vi "Set Resistor.vi"(9 "Set Resistance":T1) -> ()   [LabVIEW 2016]
uses:
  Type_defs/Resistor--enum.ctl
  USB Relay Control 256.vi
panel:
  out "USB":bool
  out "short":bool
  out "0 ohm":bool
  out "100k":bool
  out "10M":bool
  out "Gohm":bool
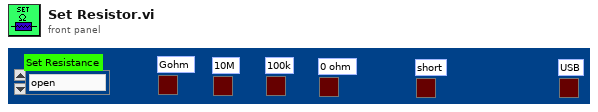
[diagram p1: front panel]
types:
  T1 = typedef "Resistor--enum.ctl" = enum16{"open", "discharge tip", "0 ohms", "100k ohm", "10M ohm", "1G ohm"}
  T2 = enum32{"invalid app kind", "Development System", "Run Time System", "Student Edition", "Embedded LabVIEW", "Evaluation", "Custom"}
  T3 = enum32{"Invalid", "Standard", "Closed", "Hidden", "Minimized", "Maximized"}
  T4 = cluster{"Core":cluster{"Current VI Reference":refnum<vi>, "Close Panel on Exit?":bool}, "Set Resistance":T1, "Previous State":u8, "Intermediate State":u8, "Final State":u8}
  T5 = cluster{"Current VI Reference":refnum<vi>, "Close Panel on Exit?":bool}
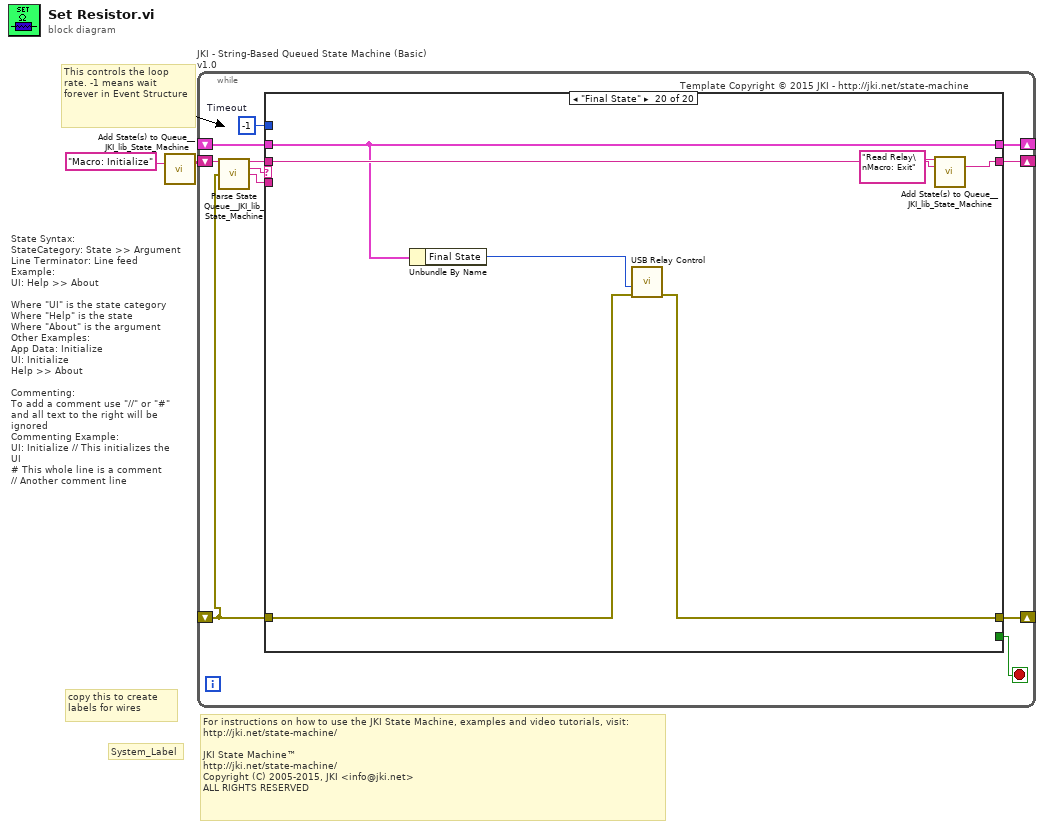
[diagram p0: block diagram]
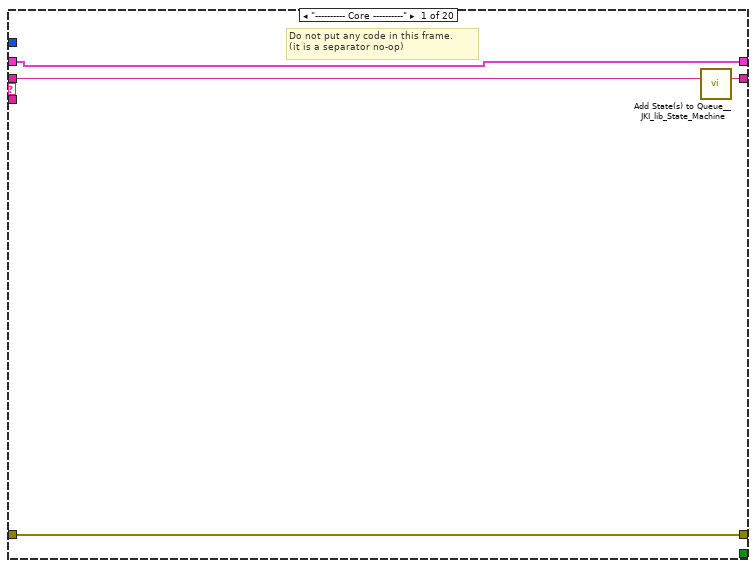
[diagram p2: hidden frame]
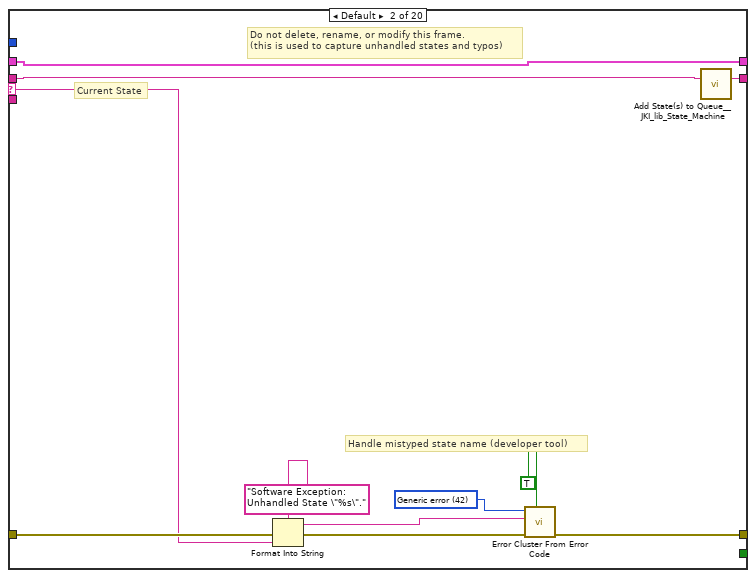
[diagram p3: hidden frame]
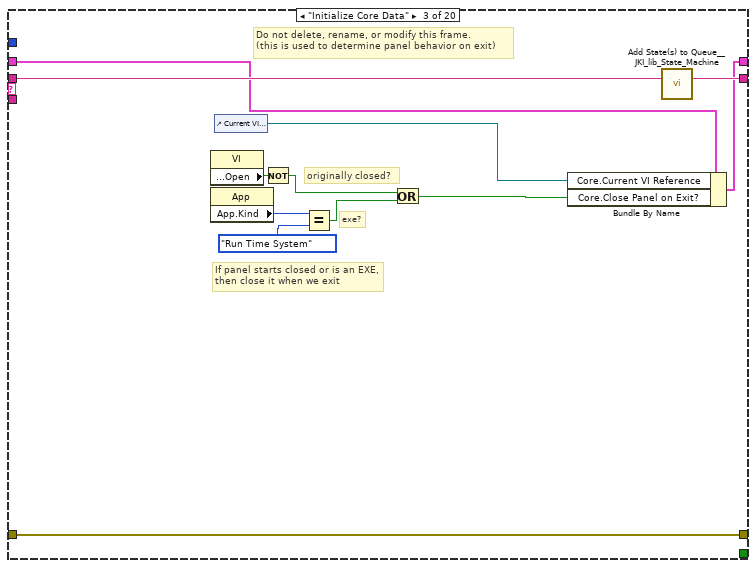
[diagram p4: hidden frame]
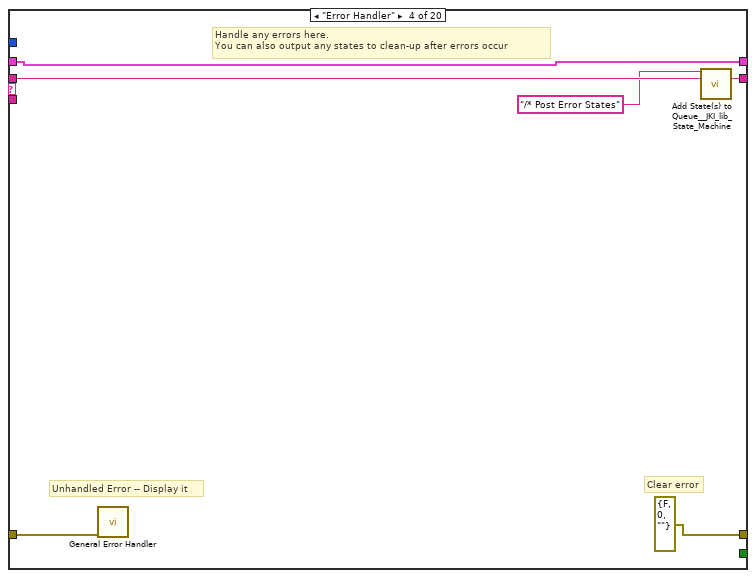
[diagram p5: hidden frame]
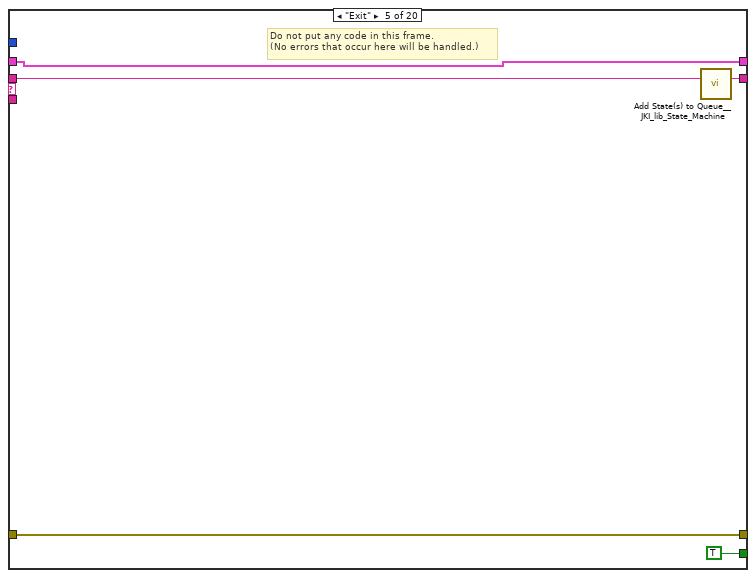
[diagram p6: hidden frame]
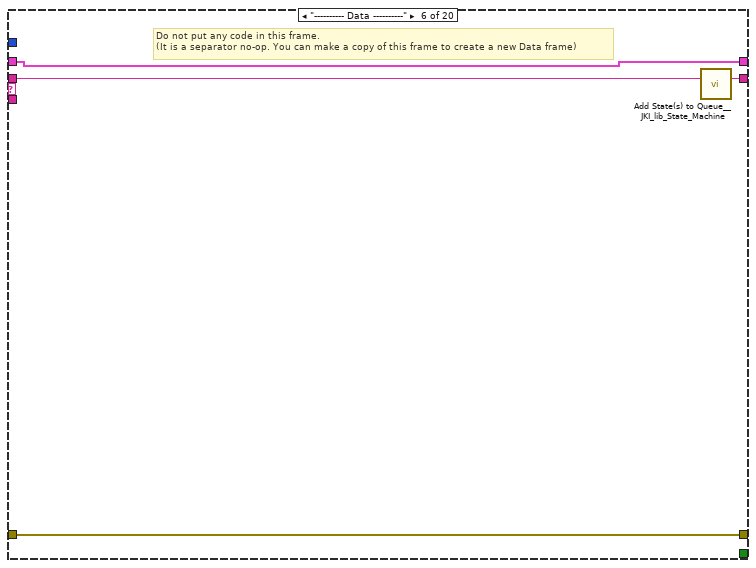
[diagram p7: hidden frame]
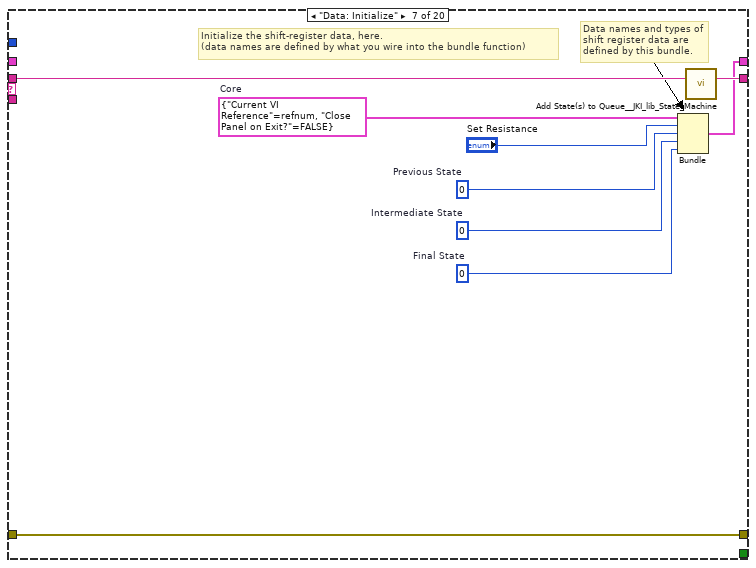
[diagram p8: hidden frame]
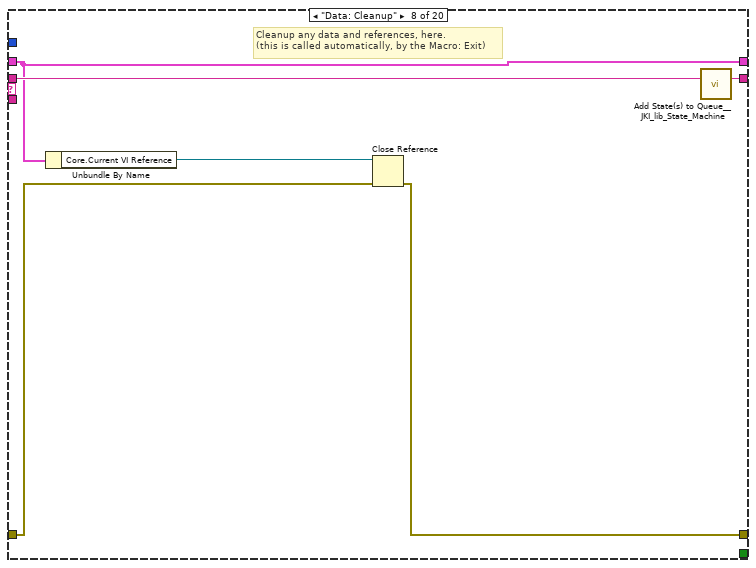
[diagram p9: hidden frame]
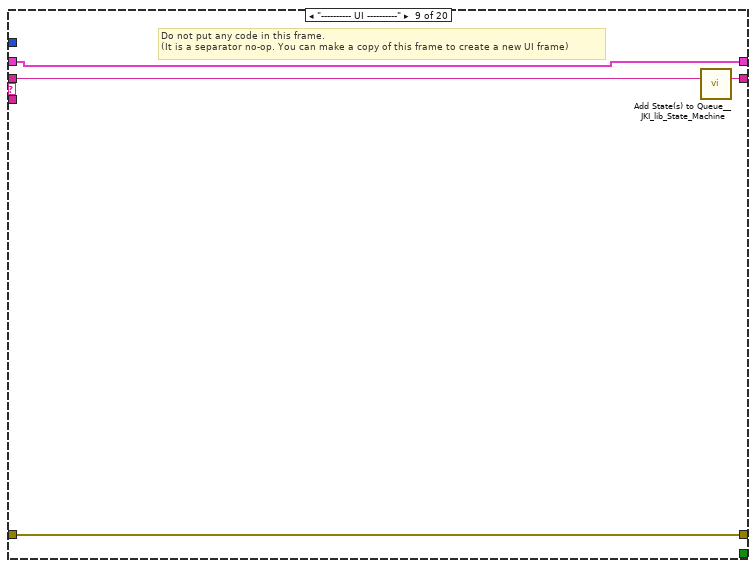
[diagram p10: hidden frame]
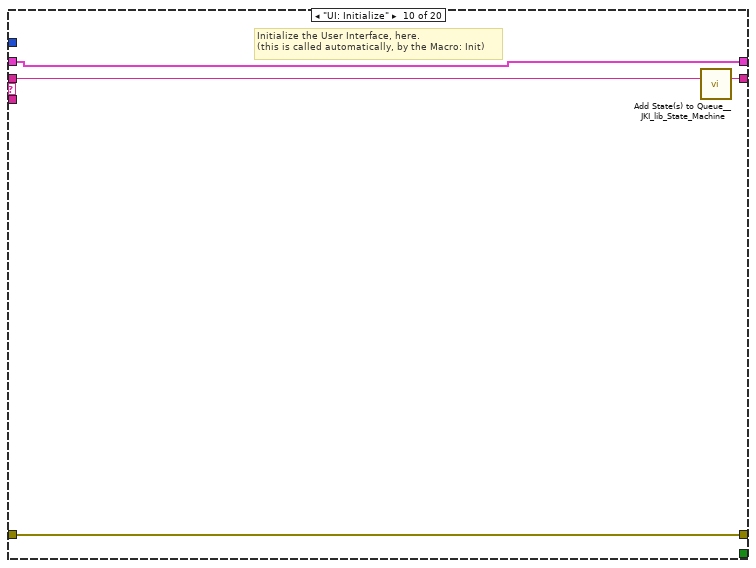
[diagram p11: hidden frame]
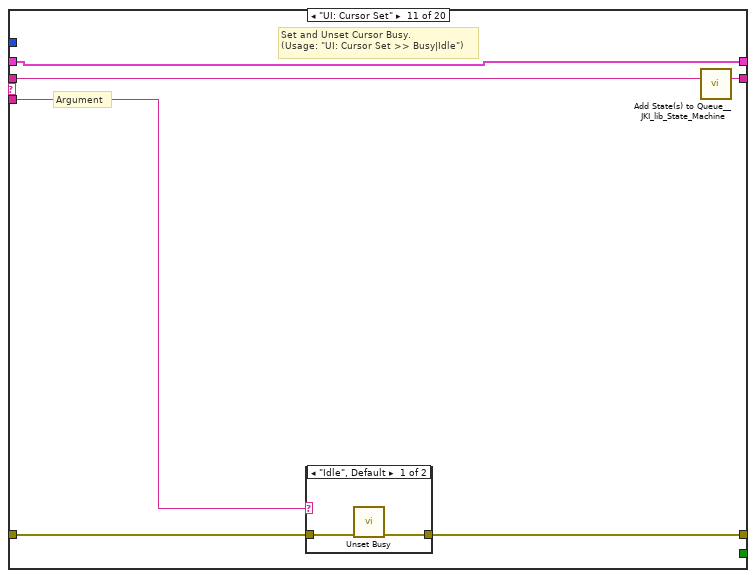
[diagram p12: hidden frame]
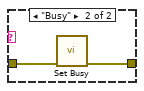
[diagram p13: hidden frame]
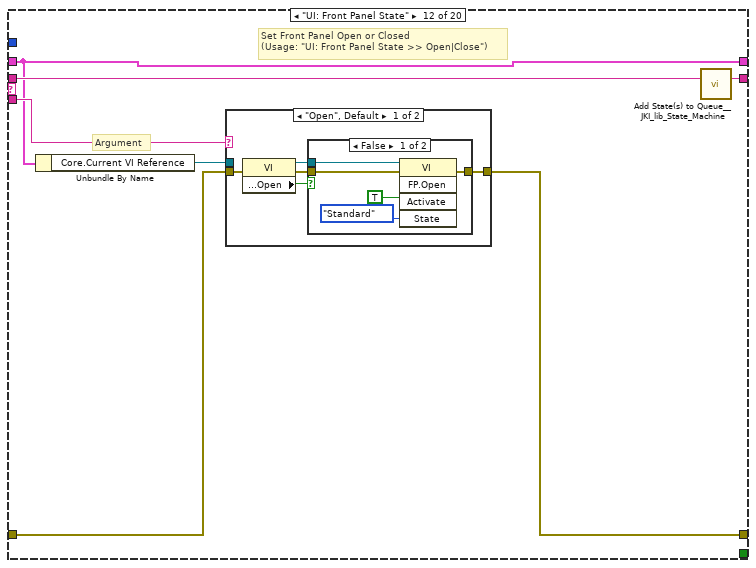
[diagram p14: hidden frame]
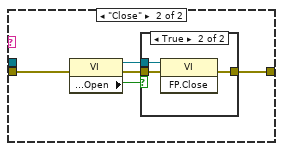
[diagram p16: hidden frame]
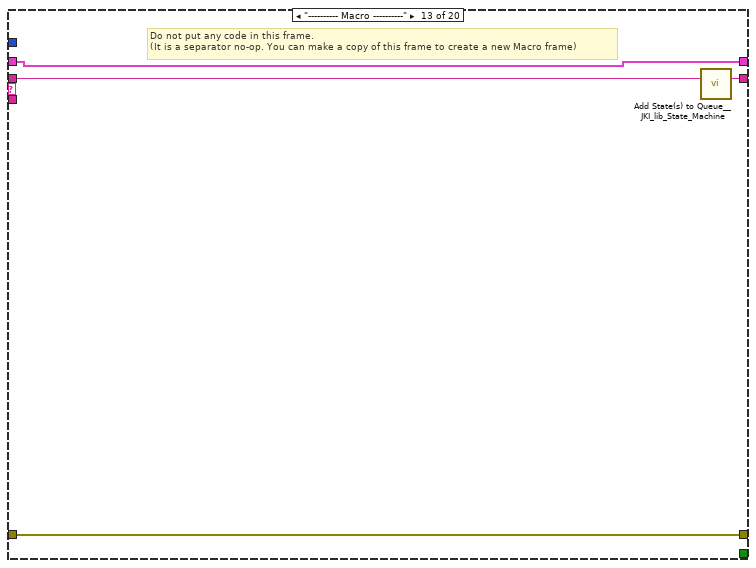
[diagram p18: hidden frame]
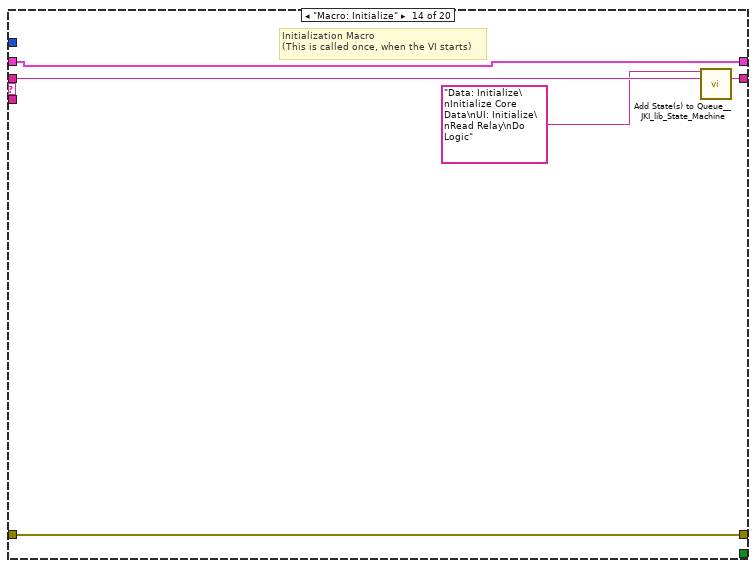
[diagram p19: hidden frame]
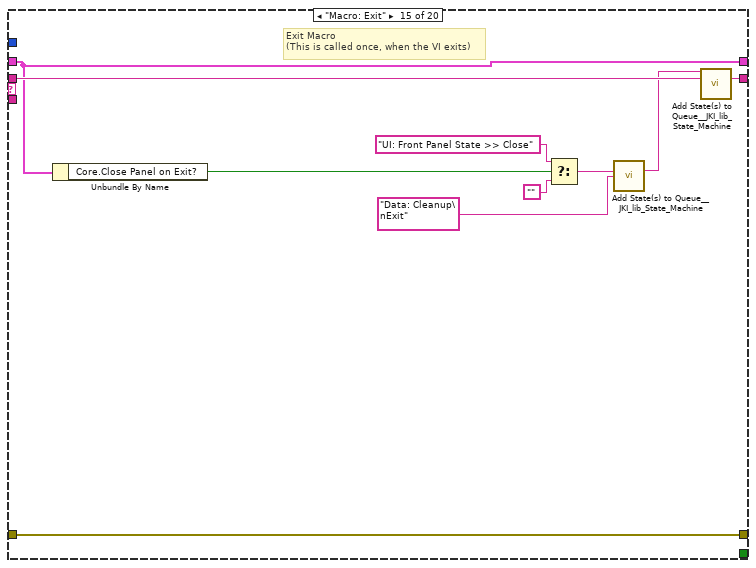
[diagram p20: hidden frame]
diagram:
  # "For instructions on how to use the JKI State Machine, examples and video tutorials, visit:\nhttp://jki.net/state-machine/\n\nJKI State Machine™\nhttp://jki.net/state-machine/\nCopyright (C) 2005-2015, JKI <info@jki.net>\nALL RIGHTS RESERVED"
  # "State Syntax:\nStateCategory: State >> Argument\nLine Terminator: Line feed\nExample:\nUI: Help >> About\n\nWhere \"UI\" is the state category\nWhere \"Help\" is the state\nWhere \"About\" is the argument\nOther Examples:\nApp Data: Initialize\nUI: Initialize\nHelp >> About\n\nCommenting:\nTo add a comment use \"//\" or \"#\" and all text to the right will be ignored\nCommenting Example:\nUI: Initialize // This initializes the UI\n# This whole line is a comment\n// Another comment line"
  # "copy this to create labels for wires"
  # "This controls the loop rate. -1 means wait forever in Event Structure"
  # "System_Label"
  n1 = call <vilib>:"Add State(s) to Queue__JKI_lib_State_Machine.vi"("State(s) in (\"\")"="Macro: Initialize") -> ("States Out"=w2:string)  [unwired: 14 in]
  n2 = while "JKI - String-Based Queued State Machine (Basic) v1.0" {
    shift-right: [w6] -> _
    shift-left: _ -> [w5]
    shift-right: [w9] -> _
    shift-left: _ -> [w3]
    shift-right: [w8] -> _
    shift-left: w2 -> [w10]
    stop <- w7 stop-if-true
    w4 = -1  # Timeout
    # "Template Copyright © 2015 JKI - http://jki.net/state-machine"
    n3 = call <vilib>:"Parse State Queue__JKI_lib_State_Machine.vi"("State Queue"=w10, "Error In (no error)"=w3) -> ("Remaining States"=w12:string, "Current State"=w13:string, "Arguments"=w11:string)  [unwired: 11 in]
    n4 = case shown="\"Final State\"" w13 {
      selector: w13 -> [_ w18 _ _ _ _ _ _ _ _ _ _ _ _ _ _ _ _ _ _]
      tunnel: w12 -> [w17 w22 w40 w46 w51 w55 w64 w70 w74 w78 w84 w95 w119 w124 w134 w138 w156 w169 w287 w294]
      tunnel: w11 -> [_ _ _ _ _ _ _ _ _ _ w79 w90 _ _ _ _ _ _ _ _]
      tunnel: w5 -> [w14 w20 w29 w43 w49 w52 _ w66 w71 w76 w82 w89 w116 w121 w126 w135 w153 w162 w285 w292]
      tunnel: [w15 w24 w38 errorcluster {"status"=FALSE, "code"=0, "source"=""} ("error out") w48 w53 w62 w67 w72 w75 w80 w92 w117 w122 w132 w136 w154 w167 w284 w290] -> w9
      tunnel: w3 -> [w15 w23 w38 w42 w48 w53 w62 w68 w72 w75 w81 w93 w117 w122 w132 w136 w154 w167 w283 w291]
      tunnel: [w16 w21 w39 w45 w50 w54 w63 w69 w73 w77 w83 w94 w118 w123 w133 w137 w155 w168 w288 w295] -> w8
      tunnel: [_ _ _ _ TRUE _ _ _ _ _ _ _ _ _ _ _ _ _ _ _] -> w7
      tunnel: [w14 w20 w30 w43 w49 w52 w59 w66 w71 w76 w82 w89 w116 w121 w126 w135 w152 w161 w285 w292] -> w6
      tunnel: w4 -> [_ _ _ _ _ _ _ _ _ _ _ _ _ _ _ _ _ _ _ _]
      frame "---------- Core ----------" {
        # "Do not put any code in this frame.\n(it is a separator no-op)"
        n5 = call <vilib>:"Add State(s) to Queue__JKI_lib_State_Machine.vi"("State(s) in (\"\")"=w17) -> ("States Out"=w16:string)  [unwired: 14 in]
      }
      frame Default {
        w27 = 42 items=["No error", "Argument error", "Memory is full", "Out of zone", "End of file", "File already open", "Generic file I/O error", "File not found", "File permission error", "Disk is full", "Duplicate path", "Too many files open", "System feature not enabled", "Resource file not found", "Cannot add resource", "Resource not found", "Image not found", "Image memory error", "Pen does not exist", "Config type invalid", "Config token not found", "Config parse error", "Config memory error", "Bad external code format", "Bad external code offset", "External code not present", "Null window", "Destroy window error", "Null menu", "Print aborted", "Bad print record", "Print driver error", "Windows error during printing", "Memory error during printing", "Print dialog error", "Generic print error", "Invalid device refnum", "Device not found", "Device parameter error", "Device unit error", "Cannot open device", "Device call aborted", "Generic error", "Cancelled by user", "Object ID too low", "Object ID too high", "Object not in heap", "Unknown heap", "Unknown object (invalid DefProc)", "Unknown object (DefProc not in table)", "Message out of range", "Invalid (null) method", "Unknown message", "Manager call not supported", "Bad address", "Network operation in progress", "Network operation timed out", "Connection is busy", "Network attribute not supported", "Network error", "Address in use", "System out of memory", "Connection aborted", "Connection refused", "Not connected", "Already connected", "Connection closed", "Initialization error (interapplication manager)", "Bad occurrence", "Wait on unbound occurrence handler", "Occurrence queue overflow", "Datalog type conflict", "Unused", "Unrecognized type (interapplication manager)", "Memory corrupt", "Failed to make temporary DLL", "Old CIN version", "Drag socket not found", "Failed to load drop-object", "Failed to register OLE object", "Failed to release OLE object", "Format specifier type mismatch", "Unknown format specifier", "Too few format specifiers", "Too many format specifiers", "Scan failed", "Newer CIN version", "Error converting to variant", "Runtime menu error", "Password tampered", "Variant attribute not found", "Incompatible variant data type", "Event data is not available", "Event Store is not present", "Occurrence is not found", "Event Queue is not created", "Event info is not available", "Refnum passed is NULL", "Error retrieving Class GUID", "Error retrieving CoClass GUID", "Error retrieving TypeLib GUID.", "Bad built application magic bytes.", "Specific driver is different from the specific driver associated with the Logical Name.", "There is no session opened to the class driver.", "Max Error", "MAX - Error with config objects", "MAX - Error loading configuration", "MAX - Group not supported"]
        # "Current State"
        # "Do not delete, rename, or modify this frame.\n(this is used to capture unhandled states and typos)"
        # "Handle mistyped state name (developer tool)"
        n6 = Format Into String(format string="Software Exception: Unhandled State \"%s\"." ("message"), error in=w23, w18) -> (resulting string=w26:string, error out=w25:errorcluster)  [unwired: 1 in]
        n7 = call <vilib>:"Error Cluster From Error Code.vi"("show call chain? (False)"=TRUE, "error in (no error)"=w25, "error message (\"\")"=w26, "error code (0)"=w27) -> ("error out"=w24:errorcluster)  [unwired: 5 in]
        n8 = call <vilib>:"Add State(s) to Queue__JKI_lib_State_Machine.vi"("State(s) in (\"\")"=w22) -> ("States Out"=w21:string)  [unwired: 14 in]
      }
      frame "Initialize Core Data" {
        # "Do not delete, rename, or modify this frame.\n(this is used to determine panel behavior on exit)"
        # "originally closed?"
        # "exe?"
        # "If panel starts closed or is an EXE, then close it when we exit"
        n9 = property class="VI"() -> ("Front Panel.Open"=w37:bool)  [unwired: 2 in, 2 out]
        n10 = property class="App"() -> ("App.Kind"=w36:T2)  [unwired: 2 in, 2 out]
        n11 = control-ref of="Current VI Reference"() -> (w31:refnum<vi>)
        n12 = Not(x=w37) -> (.not. x?=w34:bool)
        n13 = Equal?(x=w36, y=T2."Run Time System" ("Application:Kind")) -> (x = y?=w33:bool)
        n14 = Or(x=w34, y=w33) -> (x .or. y?=w32:bool)
        n15 = Bundle By Name(cluster=w29, "Core.Current VI Reference"=w31, "Core.Close Panel on Exit?"=w32) -> (w30:T4)
        n16 = call <vilib>:"Add State(s) to Queue__JKI_lib_State_Machine.vi"("State(s) in (\"\")"=w40) -> ("States Out"=w39:string)  [unwired: 14 in]
      }
      frame "Error Handler" {
        # "Unhandled Error -- Display it"
        # "Handle any errors here.\nYou can also output any states to clean-up after errors occur"
        # "Clear error"
        n17 = call <vilib>:"General Error Handler.vi"("error in (no error)"=w42) -> ()  [unwired: 10 in, 5 out]
        n18 = call <vilib>:"Add State(s) to Queue__JKI_lib_State_Machine.vi"("State(s) in Front (\"\")"="/* Post Error States", "State(s) in (\"\")"=w46) -> ("States Out"=w45:string)  [unwired: 13 in]
      }
      frame "Exit" {
        # "Do not put any code in this frame.\n(No errors that occur here will be handled.)"
        n19 = call <vilib>:"Add State(s) to Queue__JKI_lib_State_Machine.vi"("State(s) in (\"\")"=w51) -> ("States Out"=w50:string)  [unwired: 14 in]
      }
      frame "---------- Data ----------" {
        # "Do not put any code in this frame.\n(It is a separator no-op. You can make a copy of this frame to create a new Data frame)"
        n20 = call <vilib>:"Add State(s) to Queue__JKI_lib_State_Machine.vi"("State(s) in (\"\")"=w55) -> ("States Out"=w54:string)  [unwired: 14 in]
      }
      frame "Data: Initialize" {
        w56 = u8 0  # Final State
        w57 = u8 0  # Intermediate State
        w58 = u8 0  # Previous State
        w61 = T5 {"Current VI Reference"=refnum, "Close Panel on Exit?"=FALSE}  # Core
        # "Data names and types of shift register data are defined by this bundle."
        # "Initialize the shift-register data, here.\n(data names are defined by what you wire into the bundle function)"
        n21 = Bundle("Core"=w61, "Set Resistance"="Set Resistance", "Previous State"=w58, "Intermediate State"=w57, "Final State"=w56) -> (w59:T4)  [unwired: 1 in]
        n22 = call <vilib>:"Add State(s) to Queue__JKI_lib_State_Machine.vi"("State(s) in (\"\")"=w64) -> ("States Out"=w63:string)  [unwired: 14 in]
      }
      frame "Data: Cleanup" {
        # "Cleanup any data and references, here.\n(this is called automatically, by the Macro: Exit)"
        n23 = Unbundle By Name(w66) -> ("Core.Current VI Reference"=w65:refnum<vi>)
        n24 = Close Reference(reference=w65, error in (no error)=w68) -> (error out=w67:errorcluster)
        n25 = call <vilib>:"Add State(s) to Queue__JKI_lib_State_Machine.vi"("State(s) in (\"\")"=w70) -> ("States Out"=w69:string)  [unwired: 14 in]
      }
      frame "---------- UI ----------" {
        # "Do not put any code in this frame.\n(It is a separator no-op. You can make a copy of this frame to create a new UI frame)"
        n26 = call <vilib>:"Add State(s) to Queue__JKI_lib_State_Machine.vi"("State(s) in (\"\")"=w74) -> ("States Out"=w73:string)  [unwired: 14 in]
      }
      frame "UI: Initialize" {
        # "Initialize the User Interface, here.\n(this is called automatically, by the Macro: Init)"
        n27 = call <vilib>:"Add State(s) to Queue__JKI_lib_State_Machine.vi"("State(s) in (\"\")"=w78) -> ("States Out"=w77:string)  [unwired: 14 in]
      }
      frame "UI: Cursor Set" {
        # "Argument"
        # "Set and Unset Cursor Busy.\n(Usage: \"UI: Cursor Set >> Busy|Idle\")"
        n28 = case shown="\"Idle\", Default" w79 {
          tunnel: w81 -> [w86 w88]
          tunnel: [w85 w87] -> w80
          frame "Idle", Default {
            n29 = call <vilib>:"Unset Busy.vi"("error in (no error)"=w86) -> ("error out"=w85:errorcluster)  [unwired: 10 in]
          }
          frame "Busy" {
            n30 = call <vilib>:"Set Busy.vi"("error in (no error)"=w88) -> ("error out"=w87:errorcluster)  [unwired: 9 in, 1 out]
          }
        }
        n31 = call <vilib>:"Add State(s) to Queue__JKI_lib_State_Machine.vi"("State(s) in (\"\")"=w84) -> ("States Out"=w83:string)  [unwired: 14 in]
      }
      frame "UI: Front Panel State" {
        # "Argument"
        # "Set Front Panel Open or Closed\n(Usage: \"UI: Front Panel State >> Open|Close\")"
        n32 = Unbundle By Name(w89) -> ("Core.Current VI Reference"=w91:refnum<vi>)
        n33 = case shown="\"Open\", Default" w90 {
          tunnel: w93 -> [w99 w110]
          tunnel: [w100 w111] -> w92
          tunnel: w91 -> [_ _]
          frame "Open", Default {
            n34 = property class="VI"(error in=w99) -> (reference out=w97:refnum<vi>, error out=w98:errorcluster, "Front Panel.Open"=w96:bool)  [unwired: 1 in]
            n35 = case shown="False" w96 {
              tunnel: [w103 w106] -> w100
              tunnel: w98 -> [w102 w106]
              tunnel: w97 -> [w101 _]
              frame False {
                n36 = invoke class="VI" method="FP.Open"(reference=w101, error in=w102, "Activate"=TRUE, "State"=T3."Standard") -> (error out=w103:errorcluster)  [unwired: 1 in, 4 out]
              }
              frame True {
              }
            }
          }
          frame "Close" {
            n37 = property class="VI"(error in=w110) -> (reference out=w108:refnum<vi>, error out=w109:errorcluster, "Front Panel.Open"=w107:bool)  [unwired: 1 in]
            n38 = case shown="True" w107 {
              tunnel: [w112 w115] -> w111
              tunnel: w109 -> [w112 w114]
              tunnel: w108 -> [_ w113]
              frame False {
              }
              frame True {
                n39 = invoke class="VI" method="FP.Close"(reference=w113, error in=w114) -> (error out=w115:errorcluster)  [unwired: 1 in, 2 out]
              }
            }
          }
        }
        n40 = call <vilib>:"Add State(s) to Queue__JKI_lib_State_Machine.vi"("State(s) in (\"\")"=w95) -> ("States Out"=w94:string)  [unwired: 14 in]
      }
      frame "---------- Macro ----------" {
        # "Do not put any code in this frame.\n(It is a separator no-op. You can make a copy of this frame to create a new Macro frame)"
        n41 = call <vilib>:"Add State(s) to Queue__JKI_lib_State_Machine.vi"("State(s) in (\"\")"=w119) -> ("States Out"=w118:string)  [unwired: 14 in]
      }
      frame "Macro: Initialize" {
        # "Initialization Macro\n(This is called once, when the VI starts)"
        n42 = call <vilib>:"Add State(s) to Queue__JKI_lib_State_Machine.vi"("State(s) in Front (\"\")"="Data: Initialize\nInitialize Core Data\nUI: Initialize\nRead Relay\nDo Logic", "State(s) in (\"\")"=w124) -> ("States Out"=w123:string)  [unwired: 13 in]
      }
      frame "Macro: Exit" {
        # "Exit Macro\n(This is called once, when the VI exits)"
        n43 = Unbundle By Name(w126) -> ("Core.Close Panel on Exit?"=w125:bool)
        n44 = Select(t="UI: Front Panel State >> Close", s=w125, f="") -> (s? t:f=w129:string)
        n45 = call <vilib>:"Add State(s) to Queue__JKI_lib_State_Machine.vi"("State(s) in (\"\")"=w129, "State(s) at Back (\"\")"="Data: Cleanup\nExit") -> ("States Out"=w127:string)  [unwired: 13 in]
        n46 = call <vilib>:"Add State(s) to Queue__JKI_lib_State_Machine.vi"("State(s) in Front (\"\")"=w127, "State(s) in (\"\")"=w134) -> ("States Out"=w133:string)  [unwired: 13 in]
      }
      frame "---------- Relay ----------" {
        # "Template Separator\n(You can make a copy of, or modify, this frame)"
        n47 = call <vilib>:"Add State(s) to Queue__JKI_lib_State_Machine.vi"("State(s) in (\"\")"=w138) -> ("States Out"=w137:string)  [unwired: 14 in]
      }
      frame "Read Relay" {
        # "Your code here.\n(You can make a copy of, or modify, this frame)"
        n48 = call "Read_relay.vi"() -> ("unsigned 8bit integer"=w151:u8, "Boolean array"=w145:bool[])  [unwired: 1 in]
        n49 = Index Array(array=w145, index=7) -> (element=→"Gohm":bool)
        n50 = Index Array(array=w145, index=6) -> (element=→"10M":bool)
        n51 = Index Array(array=w145, index=5) -> (element=→"100k":bool)
        n52 = Index Array(array=w145, index=3) -> (element=→"0 ohm":bool)
        n53 = Index Array(array=w145, index=1) -> (element=→"short":bool)
        n54 = Bundle By Name(cluster=w153, "Previous State"=w151) -> (w152:T4)
        n55 = call <vilib>:"Add State(s) to Queue__JKI_lib_State_Machine.vi"("State(s) in (\"\")"=w156) -> ("States Out"=w155:string)  [unwired: 14 in]
        "USB" <- TRUE ("USB")
      }
      frame "Do Logic" {
        # "Your code here.\n(You can make a copy of, or modify, this frame)"
        n56 = Unbundle By Name(w162) -> ("Set Resistance"=w166:T1, "Previous State"=w157:u8)
        n57 = case shown="\"discharge tip\"" w166 {
          tunnel: [u8 0 u8 0 w179 w205 w231 w257] -> w160
          tunnel: [FALSE w173 w178 w204 w230 w256] -> w159
          tunnel: [0 2 8 32 64 128] -> w158
          tunnel: w157 -> [_ w175 w180 w206 w232 w258]
          frame "open", Default {
          }
          frame "discharge tip" {
            n58 = Not Equal?(x=w175, y=u8 0) -> (x != y?=w173:bool)
          }
          frame "0 ohms" {
            n59 = Not Equal?(x=w180, y=u8 2) -> (x != y?=w181:bool)
            n60 = case shown="True" w181 {
              tunnel: w180 -> [_ w188]
              tunnel: [u8 0 w187] -> w179
              tunnel: [TRUE w186] -> w178
              frame False {
              }
              frame True {
                n61 = Not Equal?(x=w188, y=u8 0) -> (x != y?=w189:bool)
                n62 = case shown="True" w189 {
                  tunnel: w188 -> [_ w196]
                  tunnel: [u8 8 w194] -> w187
                  tunnel: [FALSE w193] -> w186
                  frame False {
                  }
                  frame True {
                    w195 = u8 8 ("y")
                    n63 = Not Equal?(x=w196, y=w195) -> (x != y?=w197:bool)
                    n64 = case shown="False" w197 {
                      tunnel: w196 -> [_ w203]
                      tunnel: w195 -> [_ w202]
                      tunnel: [u8 8 w201] -> w194
                      tunnel: [FALSE TRUE] -> w193
                      frame False {
                      }
                      frame True {
                        n65 = Add(x=w203, y=w202) -> (x+y=w201:u8)
                      }
                    }
                  }
                }
              }
            }
          }
          frame "100k ohm" {
            n66 = Not Equal?(x=w206, y=u8 2) -> (x != y?=w207:bool)
            n67 = case shown="True" w207 {
              tunnel: w206 -> [_ w214]
              tunnel: [u8 0 w213] -> w205
              tunnel: [TRUE w212] -> w204
              frame False {
              }
              frame True {
                n68 = Not Equal?(x=w214, y=u8 0) -> (x != y?=w215:bool)
                n69 = case shown="True" w215 {
                  tunnel: w214 -> [_ w222]
                  tunnel: [u8 8 w220] -> w213
                  tunnel: [FALSE w219] -> w212
                  frame False {
                  }
                  frame True {
                    w221 = u8 32 ("y")
                    n70 = Not Equal?(x=w222, y=w221) -> (x != y?=w223:bool)
                    n71 = case shown="False" w223 {
                      tunnel: w222 -> [_ w229]
                      tunnel: w221 -> [_ w228]
                      tunnel: [u8 32 w227] -> w220
                      tunnel: [FALSE TRUE] -> w219
                      frame False {
                      }
                      frame True {
                        n72 = Add(x=w229, y=w228) -> (x+y=w227:u8)
                      }
                    }
                  }
                }
              }
            }
          }
          frame "10M ohm" {
            n73 = Not Equal?(x=w232, y=u8 2) -> (x != y?=w233:bool)
            n74 = case shown="True" w233 {
              tunnel: w232 -> [_ w240]
              tunnel: [u8 0 w239] -> w231
              tunnel: [TRUE w238] -> w230
              frame False {
              }
              frame True {
                n75 = Not Equal?(x=w240, y=u8 0) -> (x != y?=w241:bool)
                n76 = case shown="True" w241 {
                  tunnel: w240 -> [_ w248]
                  tunnel: [u8 64 w246] -> w239
                  tunnel: [FALSE w245] -> w238
                  frame False {
                  }
                  frame True {
                    w247 = u8 64 ("y")
                    n77 = Not Equal?(x=w248, y=w247) -> (x != y?=w249:bool)
                    n78 = case shown="False" w249 {
                      tunnel: w248 -> [_ w255]
                      tunnel: w247 -> [_ w254]
                      tunnel: [u8 64 w253] -> w246
                      tunnel: [FALSE TRUE] -> w245
                      frame False {
                      }
                      frame True {
                        n79 = Add(x=w255, y=w254) -> (x+y=w253:u8)
                      }
                    }
                  }
                }
              }
            }
          }
          frame "1G ohm" {
            n80 = Not Equal?(x=w258, y=u8 2) -> (x != y?=w259:bool)
            n81 = case shown="True" w259 {
              tunnel: w258 -> [_ w266]
              tunnel: [u8 0 w265] -> w257
              tunnel: [TRUE w264] -> w256
              frame False {
              }
              frame True {
                n82 = Not Equal?(x=w266, y=u8 0) -> (x != y?=w267:bool)
                n83 = case shown="True" w267 {
                  tunnel: w266 -> [_ w274]
                  tunnel: [u8 128 w272] -> w265
                  tunnel: [FALSE w271] -> w264
                  frame False {
                  }
                  frame True {
                    w273 = u8 128 ("y")
                    n84 = Not Equal?(x=w274, y=w273) -> (x != y?=w275:bool)
                    n85 = case shown="True" w275 {
                      tunnel: w274 -> [_ w281]
                      tunnel: w273 -> [_ w280]
                      tunnel: [u8 128 w279] -> w272
                      tunnel: [FALSE TRUE] -> w271
                      frame False {
                      }
                      frame True {
                        n86 = Add(x=w281, y=w280) -> (x+y=w279:u8)
                      }
                    }
                  }
                }
              }
            }
          }
        }
        n87 = Bundle By Name(cluster=w162, "Intermediate State"=w160, "Final State"=w158) -> (w161:T4)
        n88 = Select(t="Intermediate State", s=w159, f="Final State") -> (s? t:f=w165:string)
        n89 = call <vilib>:"Add State(s) to Queue__JKI_lib_State_Machine.vi"("State(s) in Front (\"\")"=w165, "State(s) in (\"\")"=w169) -> ("States Out"=w168:string)  [unwired: 13 in]
      }
      frame "Intermediate State" {
        n90 = Unbundle By Name(w285) -> ("Intermediate State"=w282:u8)
        n91 = call-poly "USB Relay Control.vi"("error in (no error)"=w283, "Send to relay board"=w282) -> ("error out"=w284:errorcluster)  [unwired: 9 in]
        n92 = call <vilib>:"Add State(s) to Queue__JKI_lib_State_Machine.vi"("State(s) in Front (\"\")"="Read Relay\nFinal State" ("State(s) in Front (\"\")"), "State(s) in (\"\")"=w287) -> ("States Out"=w288:string)  [unwired: 13 in]
      }
      frame "Final State" {
        n93 = Unbundle By Name(w292) -> ("Final State"=w289:u8)
        n94 = call-poly "USB Relay Control.vi"("error in (no error)"=w291, "Send to relay board"=w289) -> ("error out"=w290:errorcluster)  [unwired: 9 in]
        n95 = call <vilib>:"Add State(s) to Queue__JKI_lib_State_Machine.vi"("State(s) in Front (\"\")"="Read Relay\nMacro: Exit" ("State(s) in Front (\"\")"), "State(s) in (\"\")"=w294) -> ("States Out"=w295:string)  [unwired: 13 in]
      }
    }
  }
